vi "Set Index.vi"(8 "error in (no error)":errorcluster, 10 "Index":i32, 11 "Local Bus_Access in":refnum<class "Local Bus_DBL.lvclass">) -> (0 "error out":errorcluster, 3 "Local Bus_Access out":refnum<class "Local Bus_DBL.lvclass">)   [LabVIEW 2021, in "Local Bus_DBL.lvclass"]
uses:
  Local Bus_DBL.lvclass
  Local Bus_DBL.lvclass/Local Bus_DBL.ctl
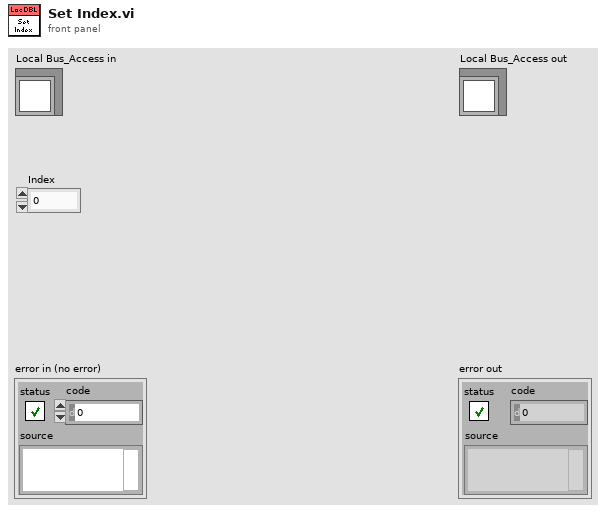
[diagram p1: front panel]
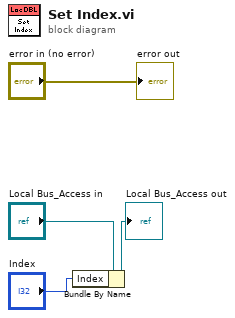
[diagram p0: block diagram]
diagram:
  n1 = Bundle By Name(cluster="Local Bus_Access in", "Index"="Index") -> (→"Local Bus_Access out":refnum<class "Local Bus_DBL.lvclass">)
  "error out" <- "error in (no error)"
